vi "RSZVB Set Renormalization Impedance.vi"(8 "error in (no error)":errorcluster {"code" format="%.0x"}, 9 "Impedance (1.0)":dbl=1.0 format="%.6f", 11 "VISA session":refnum<visa-resource-name>) -> (0 "error out":errorcluster {"code" format="%.0x"}, 3 "dup VISA session":refnum<visa-resource-name>)   [LabVIEW 2011]
doc: "Defines the target reference impedance for S-matrix export. The value is written into the file header of the generated Touchstone file. If renormalization is enabled (RSZVB Set Renormalization State.vi is set to On), it is also used for renormalization. \n\nRemote-control command(s):\nMMEMory:SETTings:RENorm:RIMPedance"
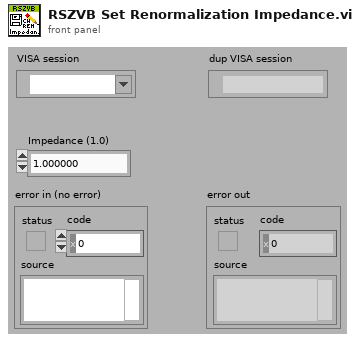
[diagram p1: front panel]
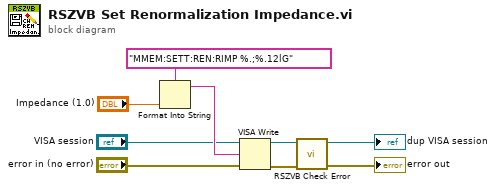
[diagram p0: block diagram]
diagram:
  n1 = Format Into String(format string="MMEM:SETT:REN:RIMP %.;%.12lG", "Impedance (1.0)") -> (resulting string=w6:string)  [unwired: 2 in, 1 out]
  n2 = VISA Write(VISA resource name="VISA session", write buffer=w6, error in (no error)="error in (no error)") -> (VISA resource name out=w8:refnum<visa-resource-name>, error out=w9:errorcluster)  [unwired: 1 out]
  n3 = call "RSZVB Check Error.vi"("error in (no error)"=w9, "VISA session"=w8) -> ("error out"=→"error out":errorcluster, "dup VISA session"=→"dup VISA session":refnum<visa-resource-name>)  [unwired: 8 in]
